vi "LSMcontroller_v66_improvedwfhandling.vi"() -> ()   [LabVIEW 2015] (continued)
                  frame #4 {
                    n2587 = call "tempconfigAO_seal.vi"("command"="get") -> ("Temp Config out"=w5912:T25)  [unwired: 1 in]
                    n2588 = Unbundle By Name(w5912) -> ("AO"=w5911:refnum<k21>[], "E_AO"=w5910:errorcluster[])
                    n2589 = call "tempconfigAI_seal.vi"("command"="get") -> ("Temp Config out"=w5899:T26)  [unwired: 1 in]
                    n2590 = call "configuration.vi"("command"="get") -> ("config out"=w5893:T11)  [unwired: 2 in, 1 out]
                    n2591 = Unbundle By Name(w5899) -> ("AI"=w5900:refnum<k21>, "E_AI"=w5901:errorcluster)
                    n2592 = Unbundle By Name(w5893) -> ("Device 1 sampleclock out"=w5890:tag, "Device 1 Starttrigger out"=w5889:tag)
                    n2593 = for {
                      tunnel: w5911 -> [w5916] mode=indexing
                      tunnel: w5910 -> [w5915] mode=indexing
                      tunnel: [w5914] -> w5906 mode=indexing
                      n2594 = call <vilib>:"DAQmx Stop Task.vi"("task/channels in"=w5916, "error in"=w5915) -> ("task out"=w5917:refnum<k21>, "error out"=w5918:errorcluster)  [unwired: 12 in]
                      n2595 = call <vilib>:"DAQmx Clear Task.vi"("task in"=w5917, "error in"=w5918) -> ("error out"=w5914:errorcluster)  [unwired: 13 in]
                    }
                    n2596 = call <vilib>:"DAQmx Stop Task.vi"("task/channels in"=w5900, "error in"=w5901) -> ("task out"=w5897:refnum<k21>, "error out"=w5896:errorcluster)  [unwired: 12 in]
                    n2597 = call <vilib>:"DAQmx Disconnect Terminals.vi"("source terminal"=tag "/Dev1/ai/SampleClock", "destination terminal"=w5890) -> ("error out"=w5887:errorcluster)  [unwired: 13 in]
                    n2598 = call <vilib>:"DAQmx Clear Task.vi"("task in"=w5897, "error in"=w5896) -> ("error out"=w5895:errorcluster)  [unwired: 13 in]
                    n2599 = call "tempconfigAO_seal.vi"("command"="get") -> ("Temp Config out"=w5907:T25)  [unwired: 1 in]
                    n2600 = Bundle By Name(cluster=w5907, "E_AO"=w5906) -> (w5905:T25)
                    n2601 = call "tempconfigAI_seal.vi"("command"="get") -> ("Temp Config out"=w5903:T26)  [unwired: 1 in]
                    n2602 = Bundle By Name(cluster=w5903, "E_AI"=w5895) -> (w5894:T26)
                    n2603 = call "tempconfigAO_seal.vi"("Temp Config in"=w5905, "command"="set") -> ()  [unwired: 1 out]
                    n2604 = call "tempconfigAI_seal.vi"("Temp Config in"=w5894, "command"="set") -> ()  [unwired: 1 out]
                    n2605 = call <vilib>:"DAQmx Disconnect Terminals.vi"("source terminal"=tag "/Dev1/ai/StartTrigger", "destination terminal"=w5889, "error in"=w5887) -> ()  [unwired: 12 in, 1 out]
                  }
                  frame #5 {
                    n2606 = call "zeropatch.vi"() -> ()  [unwired: 12 in]
                  }
                  frame #6 {
                    w5922 = T21 4 items=["no dialog", "OK message", "continue or stop message", "OK message + warnings", "continue/stop + warnings"] ("type of dialog (OK msg:1)")
                    n2607 = call "displayerrors.vi"() -> ("error IO"=w5921:errorcluster)
                    n2608 = call <vilib>:"Simple Error Handler.vi"("type of dialog (OK msg:1)"=w5922, "error in (no error)"=w5921) -> ("error out"=w5920:errorcluster)  [unwired: 3 in, 4 out]
                    n2609 = call <vilib>:"Clear Errors.vi"("error in (no error)"=w5920) -> ("error out"=w5919:errorcluster)  [unwired: 5 in, 1 out]
                    n2610 = call "seterrors.vi"("error IO"=w5919) -> ()
                  }
                }
              }
            }
          }
          event "readpatch": Value Change {
            n2611 = event-data() -> ()  [unwired: 1 in, 6 out]
            n2612 = local read "readpatch"() -> (w5923:bool)
            n2613 = case shown="True" w5923 {
              frame False {
              }
              frame True {
                n2614 = stacked-sequence {
                  seq-local: [w5924 _ _ _ _ _] -> [_ w5957 _ w6009 _ _]
                  frame #0 {
                    n2615 = stacked-sequence {
                      tunnel: [_ w5936 _] -> w5924
                      frame #0 {
                        n2616 = call "2pparameters.vi"("command"="get") -> ("params out"=w5929:T10)  [unwired: 1 in]
                        n2617 = Unbundle By Name(w5929) -> ("autoshutter"=w5930:bool)
                        n2618 = local read "OCchecked?"() -> (w5927:bool)
                        n2619 = call "sealtestwfparams.vi"("command"="set") -> ()  [unwired: 6 in, 1 out]
                        n2620 = case shown="False" w5927 {
                          frame False {
                            n2621 = One Button Dialog(message="Is the OC gain correct?", button name ("OK")="ok") -> (true=w5931:bool)
                            n2622 = local write "OCchecked?"(w5931) -> ()
                          }
                          frame True {
                          }
                        }
                        n2623 = case shown="True" w5930 {
                          frame False {
                          }
                          frame True {
                            n2624 = call "shuttercontrol.vi"("command"="close") -> ()  [unwired: 1 in, 1 out]
                          }
                        }
                        n2625 = call "allAI-temp.vi"("command"=enum16{"get", "set", "clear", "append"}."clear") -> ()  [unwired: 3 in, 2 out]
                      }
                      frame #1 {
                        n2626 = call "sealtestwfparams.vi"("command"="get") -> ("Params out"=w5942:T22)  [unwired: 6 in]
                        n2627 = Unbundle By Name(w5942) -> ("AO parameters"=w5940:T23)
                        n2628 = Index Array(array=w5940, index=1) -> (element=w5939:T24)
                        n2629 = call "generateRampedSquareWave_fromAOparameters.vi"("AO params"=w5939) -> ("Waveform"=w5935:waveform(dbl), "wflength"=w5936:i32)
                        n2630 = Build Array(w5935) -> (w5938:waveform(dbl)[])
                        n2631 = call "waveformssealtestbuffer.vi"("AO wf in"=w5938, "command"="set") -> ()  [unwired: 1 out]
                      }
                      frame #2 {
                        n2632 = local read "Vholding (mV)"() -> (w5945:sgl)
                        n2633 = local read "Current Clamp"() -> (w5951:bool)
                        n2634 = local read "Voltage Clamp"() -> (w5950:bool)
                        n2635 = local read "OCgain"() -> (w5946:sgl)
                        n2636 = local read "CC_ICgain"() -> (w5949:dbl)
                        n2637 = local read "holdon"() -> (w5944:bool)
                        n2638 = call "patchparameters.vi"("command"="get") -> ("Params out"=w5953:T13)  [unwired: 1 in]
                        n2639 = Bundle By Name(cluster=w5953, "VC"=w5950, "CC"=w5951, "CC_icg (pA/mv)"=w5949, "VC_icg (mV/mV)"=10.0, "OCG (mV/pA)"=w5946, "OVG (mV/mV)"=0.1, "Vhold (mV)"=w5945, "holdon"=w5944) -> (w5952:T13)
                        n2640 = call "patchparameters.vi"("Params in"=w5952, "command"="set") -> ()  [unwired: 1 out]
                      }
                    }
                  }
                  frame #1 {
                    w5956 = 2
                    n2641 = call "patchparameters.vi"("command"="get") -> ("Params out"=w5964:T13)  [unwired: 1 in]
                    n2642 = Unbundle By Name(w5964) -> ("holdon"=w5963:bool, "Vhold (mV)"=w5962:sgl, "CC_icg (pA/mv)"=w5970:sgl, "CC"=w5968:bool, "VC_icg (mV/mV)"=w5969:sgl)
                    n2643 = Select(t=w5970, s=w5968, f=w5969) -> (s? t:f=w5971:sgl)
                    n2644 = To Single Precision Float(number=0.001 ("y")) -> (single precision float=w5972:sgl)
                    n2645 = Compound Arithmetic op=MULTIPLY(w5962, w5971, w5972) -> (w5966:sgl)
                    n2646 = case shown="False" w5963 {
                      tunnel: w5966 -> [_ w5984]
                      tunnel: [0.0 w5984] -> w5959
                      frame False {
                      }
                      frame True {
                      }
                    }
                    n2647 = Greater Than 0?(x=w5956) -> (x > 0?=w5958:bool)
                    n2648 = case shown="True" w5958 {
                      tunnel: w5957 -> [_ w5973]
                      tunnel: w5956 -> [_ w5976]
                      frame False {
                      }
                      frame True {
                        n2649 = Initialize Array(sgl 0.0 ("element"), w5976, w5973) -> (w5974:sgl[][])
                        n2650 = call "allAI-temp.vi"("array in"=w5974, "command"=enum16{"get", "set", "clear", "append"}."set") -> ()  [unwired: 2 in, 2 out]
                      }
                    }
                    n2651 = flat-sequence {
                      tunnel: w5957 -> [w5980]
                      tunnel: w5957 -> [w5979]
                      tunnel: [w5979] -> w5961
                      tunnel: [w5978] -> w5960
                      tunnel: w5959 -> [w5978]
                      tunnel: w5961 -> [w5982]
                      tunnel: w5960 -> [w5981]
                      frame #0 {
                        n2652 = call "prepAI_sealtest.vi"("samples per channel"=w5980) -> ()  [unwired: 2 in]
                      }
                      frame #1 {
                        n2653 = call "prepAO_sealtest.vi"("Vhold"=w5981, "samples per channel"=w5982) -> ()  [unwired: 1 in]
                      }
                    }
                  }
                  frame #2 {
                    n2654 = stacked-sequence {
                      frame #0 {
                        n2655 = call "tempconfigAO.vi"("command"="get") -> ("Temp Config out"=w5988:T25)  [unwired: 1 in]
                        n2656 = Unbundle By Name(w5988) -> ("AO"=w5989:refnum<k21>[], "E_AO"=w5990:errorcluster[])
                        n2657 = for {
                          tunnel: w5989 -> [w5998] mode=indexing
                          tunnel: w5990 -> [w5997] mode=indexing
                          tunnel: [w5996] -> w5992 mode=indexing
                          tunnel: [w5995] -> w5993 mode=indexing
                          n2658 = call <vilib>:"DAQmx Start Task.vi"("task/channels in"=w5998, "error in"=w5997) -> ("task out"=w5996:refnum<k21>, "error out"=w5995:errorcluster)  [unwired: 12 in]
                        }
                        n2659 = call "tempconfigAO.vi"("command"="get") -> ("Temp Config out"=w5991:T25)  [unwired: 1 in]
                        n2660 = Bundle By Name(cluster=w5991, "AO"=w5992, "E_AO"=w5993) -> (w5994:T25)
                        n2661 = call "tempconfigAO.vi"("Temp Config in"=w5994, "command"="set") -> ()  [unwired: 1 out]
                      }
                      frame #1 {
                        n2662 = call "tempconfigAI.vi"("command"="get") -> ("Temp Config out"=w6000:T26)  [unwired: 1 in]
                        n2663 = Unbundle By Name(w6000) -> ("AI"=w6005:refnum<k21>, "E_AI"=w6006:errorcluster)
                        n2664 = call <vilib>:"DAQmx Start Task.vi"("task/channels in"=w6005, "error in"=w6006) -> ("task out"=w6007:refnum<k21>, "error out"=w6008:errorcluster)  [unwired: 12 in]
                        n2665 = call "tempconfigAI.vi"("command"="get") -> ("Temp Config out"=w6002:T26)  [unwired: 1 in]
                        n2666 = Bundle By Name(cluster=w6002, "AI"=w6007, "E_AI"=w6008) -> (w6004:T26)
                        n2667 = call "tempconfigAI.vi"("Temp Config in"=w6004, "command"="set") -> ()  [unwired: 1 out]
                      }
                    }
                  }
                  frame #3 {
                    n2668 = while {
                      tunnel: w6009 -> [w6010]
                      stop <- w6011 stop-if-true
                      n2669 = local read "readpatch"() -> (w6014:bool)
                      n2670 = Not(x=w6014) -> (.not. x?=w6013:bool)
                      n2671 = case shown="True" w6013 {
                        tunnel: w6010 -> [w6015 _]
                        frame False {
                          n2672 = stacked-sequence {
                            seq-local: [w6016 _ _ _ _ _] -> [_ w6025 _ w6048 w6095 w6114]
                            tunnel: w6015 -> [_ _ w6033 _ w6094 _]
                            frame #0 {
                              n2673 = call "patchparameters.vi"("command"="get") -> ("Params out"=w6023:T13)  [unwired: 1 in]
                              n2674 = local read "Vholding (mV)"() -> (w6020:sgl)
                              n2675 = Unbundle By Name(w6023) -> ("Vhold (mV)"=w6019:sgl, "holdon"=w6022:bool)
                              n2676 = local read "holdon"() -> (w6021:bool)
                              n2677 = Not Equal?(x=w6020, y=w6019) -> (x != y?=w6018:bool)
                              n2678 = Not Equal?(x=w6022, y=w6021) -> (x != y?=w6017:bool)
                              n2679 = Or(x=w6018, y=w6017) -> (x .or. y?=w6016:bool)
                            }
                            frame #1 {
                              n2680 = case shown="False" w6025 {
                                frame False {
                                }
                                frame True {
                                n2681 = local read "Vholding (mV)"() -> (w6028:sgl)
                                n2682 = local read "holdon"() -> (w6026:bool)
                                n2683 = call "patchparameters.vi"("command"="get") -> ("Params out"=w6029:T13)  [unwired: 1 in]
                                n2684 = Bundle By Name(cluster=w6029, "Vhold (mV)"=w6028, "holdon"=w6026) -> (w6027:T13)
                                n2685 = call "patchparameters.vi"("Params in"=w6027, "command"="set") -> ()  [unwired: 1 out]
                                }
                              }
                            }
                            frame #2 {
                              n2686 = call "tempconfigAI.vi"("command"="get") -> ("Temp Config out"=w6043:T26)  [unwired: 1 in]
                              n2687 = Unbundle By Name(w6043) -> ("AI"=w6042:refnum<k21>, "E_AI"=w6041:errorcluster)
                              n2688 = call-poly <vilib>:"DAQmx Read.vi"("task/channels in"=w6042, "number of samples per channel"=w6033, "timeout"=10.0, "error in"=w6041) -> ("task out"=w6037:refnum<k21>, "data"=w6034:i16[][], "error out"=w6046:errorcluster)  [unwired: 9 in]
                              n2689 = call "tempconfigAI.vi"("command"="get") -> ("Temp Config out"=w6038:T26)  [unwired: 1 in]
                              n2690 = Bundle By Name(cluster=w6038, "AI"=w6037, "E_AI"=w6046) -> (w6045:T26)
                              n2691 = To Single Precision Float(number=w6034) -> (single precision float=w6036:sgl[][])
                              n2692 = call "tempconfigAI.vi"("Temp Config in"=w6045, "command"="set") -> ()  [unwired: 1 out]
                              n2693 = call "allAI-temp.vi"("array in"=w6036, "command"=enum16{"get", "set", "clear", "append"}."set") -> ()  [unwired: 2 in, 2 out]
                            }
                            frame #3 {
                              n2694 = case shown="True" w6048 {
                                frame False {
                                }
                                frame True {
                                n2695 = call "tempconfigAO.vi"("command"="get") -> ("Temp Config out"=w6087:T25)  [unwired: 1 in]
                                n2696 = Unbundle By Name(w6087) -> ("AO"=w6086:refnum<k21>[], "E_AO"=w6085:errorcluster[])
                                n2697 = call "tempconfigAI.vi"("command"="get") -> ("Temp Config out"=w6074:T26)  [unwired: 1 in]
                                n2698 = Unbundle By Name(w6074) -> ("AI"=w6075:refnum<k21>, "E_AI"=w6076:errorcluster)
                                n2699 = for {
                                tunnel: w6086 -> [w6091] mode=indexing
                                tunnel: w6085 -> [w6090] mode=indexing
                                tunnel: [w6089] -> w6081 mode=indexing
                                n2700 = call <vilib>:"DAQmx Stop Task.vi"("task/channels in"=w6091, "error in"=w6090) -> ("task out"=w6092:refnum<k21>, "error out"=w6093:errorcluster)  [unwired: 12 in]
                                n2701 = call <vilib>:"DAQmx Clear Task.vi"("task in"=w6092, "error in"=w6093) -> ("error out"=w6089:errorcluster)  [unwired: 13 in]
                                }
                                n2702 = call <vilib>:"DAQmx Stop Task.vi"("task/channels in"=w6075, "error in"=w6076) -> ("task out"=w6072:refnum<k21>, "error out"=w6071:errorcluster)  [unwired: 12 in]
                                n2703 = call <vilib>:"DAQmx Clear Task.vi"("task in"=w6072, "error in"=w6071) -> ("error out"=w6070:errorcluster)  [unwired: 13 in]
                                n2704 = call "tempconfigAO.vi"("command"="get") -> ("Temp Config out"=w6082:T25)  [unwired: 1 in]
                                n2705 = Bundle By Name(cluster=w6082, "E_AO"=w6081) -> (w6080:T25)
                                n2706 = call "tempconfigAI.vi"("command"="get") -> ("Temp Config out"=w6078:T26)  [unwired: 1 in]
                                n2707 = Bundle By Name(cluster=w6078, "E_AI"=w6070) -> (w6069:T26)
                                n2708 = call "tempconfigAO.vi"("Temp Config in"=w6080, "command"="set") -> ()  [unwired: 1 out]
                                n2709 = call "tempconfigAI.vi"("Temp Config in"=w6069, "command"="set") -> ()  [unwired: 1 out]
                                }
                              }
                              n2710 = call "allAI-temp.vi"("command"=enum16{"get", "set", "clear", "append"}."get") -> ("array out"=w6052:sgl[][])  [unwired: 3 in, 1 out]
                              n2711 = call "tempconfigAI.vi"("command"="get") -> ("Temp Config out"=w6064:T26)  [unwired: 1 in]
                              n2712 = call "tempconfigAI.vi"("command"="get") -> ("Temp Config out"=w6066:T26)  [unwired: 1 in]
                              n2713 = Unbundle By Name(w6064) -> ("header"=w6062:dbl[])
                              n2714 = Unbundle By Name(w6066) -> ("header"=w6068:dbl[])
                              n2715 = Index Array(array=w6052, index (row) #1=1 ("index (row)"), index (row) #2=0 ("index (row)")) -> (element #1=w6050:sgl[], element #2=w6049:sgl[])  [unwired: 2 in]
                              n2716 = local read "OCgain"() -> (w6056:sgl)
                              n2717 = call "Unscaledtoscaled.vi"("Unscaled Data"=w6050, "Header Information"=w6062) -> ("Array"=w6061:sgl[])  [unwired: 1 in]
                              n2718 = call "Unscaledtoscaled.vi"("Unscaled Data"=w6049, "Header Information"=w6068) -> ("Array"=w6065:sgl[])  [unwired: 1 in]
                              n2719 = Multiply(x=w6061, y=0.1) -> (x*y=w6058:dbl[])
                              n2720 = Divide(x=w6065, y=w6056) -> (x/y=w6057:sgl[])
                              n2721 = Build Array(w6058, w6057) -> (w6060:dbl[][])
                              n2722 = Multiply(x=w6060, y=1000.0) -> (x*y=w6047:dbl[][])
                              n2723 = local write "Patch readout"(w6047) -> ()
                            }
                            frame #4 {
                              n2724 = case shown="True" w6095 {
                                tunnel: w6094 -> [_ w6096]
                                frame False {
                                }
                                frame True {
                                n2725 = call "patchparameters.vi"("command"="get") -> ("Params out"=w6100:T13)  [unwired: 1 in]
                                n2726 = Unbundle By Name(w6100) -> ("holdon"=w6099:bool, "Vhold (mV)"=w6098:sgl, "CC_icg (pA/mv)"=w6106:sgl, "CC"=w6104:bool, "VC_icg (mV/mV)"=w6105:sgl)
                                n2727 = Select(t=w6106, s=w6104, f=w6105) -> (s? t:f=w6107:sgl)
                                n2728 = To Single Precision Float(number=0.001 ("y")) -> (single precision float=w6108:sgl)
                                n2729 = Compound Arithmetic op=MULTIPLY(w6098, w6107, w6108) -> (w6102:sgl)
                                n2730 = case shown="True" w6099 {
                                tunnel: w6102 -> [_ w6113]
                                tunnel: [0.0 w6113] -> w6097
                                frame False {
                                }
                                frame True {
                                }
                                }
                                n2731 = flat-sequence {
                                tunnel: w6096 -> [w6109]
                                tunnel: w6097 -> [w6111]
                                tunnel: w6096 -> [w6110]
                                frame #0 {
                                n2732 = call "prepAI_sealtest.vi"("samples per channel"=w6109) -> ()  [unwired: 2 in]
                                }
                                frame #1 {
                                n2733 = call "prepAO_sealtest.vi"("Vhold"=w6111, "samples per channel"=w6110) -> ()  [unwired: 1 in]
                                }
                                }
                                }
                              }
                            }
                            frame #5 {
                              n2734 = case shown="True" w6114 {
                                frame False {
                                }
                                frame True {
                                n2735 = stacked-sequence {
                                frame #0 {
                                n2736 = call "tempconfigAO.vi"("command"="get") -> ("Temp Config out"=w6121:T25)  [unwired: 1 in]
                                n2737 = Unbundle By Name(w6121) -> ("AO"=w6120:refnum<k21>[], "E_AO"=w6119:errorcluster[])
                                n2738 = for {
                                tunnel: w6120 -> [w6128] mode=indexing
                                tunnel: w6119 -> [w6127] mode=indexing
                                tunnel: [w6126] -> w6117 mode=indexing
                                tunnel: [w6125] -> w6116 mode=indexing
                                n2739 = call <vilib>:"DAQmx Start Task.vi"("task/channels in"=w6128, "error in"=w6127) -> ("task out"=w6126:refnum<k21>, "error out"=w6125:errorcluster)  [unwired: 12 in]
                                }
                                n2740 = call "tempconfigAO.vi"("command"="get") -> ("Temp Config out"=w6118:T25)  [unwired: 1 in]
                                n2741 = Bundle By Name(cluster=w6118, "AO"=w6117, "E_AO"=w6116) -> (w6115:T25)
                                n2742 = call "tempconfigAO.vi"("Temp Config in"=w6115, "command"="set") -> ()  [unwired: 1 out]
                                }
                                frame #1 {
                                n2743 = call "tempconfigAI.vi"("command"="get") -> ("Temp Config out"=w6130:T26)  [unwired: 1 in]
                                n2744 = Unbundle By Name(w6130) -> ("AI"=w6135:refnum<k21>, "E_AI"=w6136:errorcluster)
                                n2745 = call <vilib>:"DAQmx Start Task.vi"("task/channels in"=w6135, "error in"=w6136) -> ("task out"=w6137:refnum<k21>, "error out"=w6138:errorcluster)  [unwired: 12 in]
                                n2746 = call "tempconfigAI.vi"("command"="get") -> ("Temp Config out"=w6132:T26)  [unwired: 1 in]
                                n2747 = Bundle By Name(cluster=w6132, "AI"=w6137, "E_AI"=w6138) -> (w6134:T26)
                                n2748 = call "tempconfigAI.vi"("Temp Config in"=w6134, "command"="set") -> ()  [unwired: 1 out]
                                }
                                }
                                }
                              }
                            }
                          }
                        }
                        frame True {
                        }
                      }
                      n2749 = local read "readpatch"() -> (w6012:bool)
                      n2750 = Not(x=w6012) -> (.not. x?=w6011:bool)
                    }
                  }
                  frame #4 {
                    n2751 = call "tempconfigAO.vi"("command"="get") -> ("Temp Config out"=w6164:T25)  [unwired: 1 in]
                    n2752 = Unbundle By Name(w6164) -> ("AO"=w6163:refnum<k21>[], "E_AO"=w6162:errorcluster[])
                    n2753 = call "configuration.vi"("command"="get") -> ("config out"=w6145:T11)  [unwired: 2 in, 1 out]
                    n2754 = call "tempconfigAI.vi"("command"="get") -> ("Temp Config out"=w6151:T26)  [unwired: 1 in]
                    n2755 = Unbundle By Name(w6145) -> ("Device 1 sampleclock out"=w6142:tag, "Device 1 Starttrigger out"=w6141:tag)
                    n2756 = Unbundle By Name(w6151) -> ("AI"=w6152:refnum<k21>, "E_AI"=w6153:errorcluster)
                    n2757 = for {
                      tunnel: w6163 -> [w6168] mode=indexing
                      tunnel: w6162 -> [w6167] mode=indexing
                      tunnel: [w6166] -> w6158 mode=indexing
                      n2758 = call <vilib>:"DAQmx Stop Task.vi"("task/channels in"=w6168, "error in"=w6167) -> ("task out"=w6169:refnum<k21>, "error out"=w6170:errorcluster)  [unwired: 12 in]
                      n2759 = call <vilib>:"DAQmx Clear Task.vi"("task in"=w6169, "error in"=w6170) -> ("error out"=w6166:errorcluster)  [unwired: 13 in]
                    }
                    n2760 = call <vilib>:"DAQmx Stop Task.vi"("task/channels in"=w6152, "error in"=w6153) -> ("task out"=w6149:refnum<k21>, "error out"=w6148:errorcluster)  [unwired: 12 in]
                    n2761 = call <vilib>:"DAQmx Disconnect Terminals.vi"("source terminal"=tag "/Dev1/ai/SampleClock", "destination terminal"=w6142) -> ("error out"=w6139:errorcluster)  [unwired: 13 in]
                    n2762 = call <vilib>:"DAQmx Clear Task.vi"("task in"=w6149, "error in"=w6148) -> ("error out"=w6147:errorcluster)  [unwired: 13 in]
                    n2763 = call "tempconfigAO.vi"("command"="get") -> ("Temp Config out"=w6159:T25)  [unwired: 1 in]
                    n2764 = Bundle By Name(cluster=w6159, "E_AO"=w6158) -> (w6157:T25)
                    n2765 = call "tempconfigAI.vi"("command"="get") -> ("Temp Config out"=w6155:T26)  [unwired: 1 in]
                    n2766 = Bundle By Name(cluster=w6155, "E_AI"=w6147) -> (w6146:T26)
                    n2767 = call "tempconfigAO.vi"("Temp Config in"=w6157, "command"="set") -> ()  [unwired: 1 out]
                    n2768 = call <vilib>:"DAQmx Disconnect Terminals.vi"("source terminal"=tag "/Dev1/ai/StartTrigger", "destination terminal"=w6141, "error in"=w6139) -> ()  [unwired: 12 in, 1 out]
                    n2769 = call "tempconfigAI.vi"("Temp Config in"=w6146, "command"="set") -> ()  [unwired: 1 out]
                  }
                  frame #5 {
                    w6173 = T21 4 items=["no dialog", "OK message", "continue or stop message", "OK message + warnings", "continue/stop + warnings"] ("type of dialog (OK msg:1)")
                    n2770 = call "displayerrors.vi"() -> ("error IO"=w6172:errorcluster)
                    n2771 = call "zeropatch.vi"() -> ()  [unwired: 12 in]
                    n2772 = call <vilib>:"Simple Error Handler.vi"("type of dialog (OK msg:1)"=w6173, "error in (no error)"=w6172) -> ("error out"=w6171:errorcluster)  [unwired: 3 in, 4 out]
                    n2773 = call <vilib>:"Clear Errors.vi"("error in (no error)"=w6171) -> ()  [unwired: 5 in, 2 out]
                  }
                }
              }
            }
          }
          event "Current Clamp": Value Change {
            n2774 = event-data() -> ()  [unwired: 1 in, 6 out]
            n2775 = local read "Current Clamp"() -> (w6178:bool)
            n2776 = property on="Vholding (mV)" class="DigNum (strict)"("Caption.Text"="Ihold (pA)") -> ()  [unwired: 2 in, 2 out]
            n2777 = Not(x=w6178) -> (.not. x?=w6177:bool)
            n2778 = property on="Voltage Clamp" class="Bool (strict)"("Value"=w6177) -> ()  [unwired: 2 in, 2 out]
            n2779 = One Button Dialog(message="Have you switched the HEKA to CC and changed the external input cable?", button name ("OK")="Ok") -> ()  [unwired: 1 out]
          }
          event "Voltage Clamp": Value Change {
            n2780 = event-data() -> ()  [unwired: 1 in, 6 out]
            n2781 = local read "Voltage Clamp"() -> (w6183:bool)
            n2782 = Not(x=w6183) -> (.not. x?=w6182:bool)
            n2783 = property on="Current Clamp" class="Bool (strict)"("Value"=w6182) -> ()  [unwired: 2 in, 2 out]
            n2784 = One Button Dialog(message="Have you switched the HEKA to VC and changed the external input cable?", button name ("OK")="Ok") -> ()  [unwired: 1 out]
            n2785 = property on="Vholding (mV)" class="DigNum (strict)"("Caption.Text"="Vhold (mV)") -> ()  [unwired: 2 in, 2 out]
          }
          event "OCgain": Value Change {
            n2786 = event-data() -> ()  [unwired: 1 in, 6 out]
            n2787 = local read "OCgain"() -> (w6186:sgl)
            n2788 = Less?(x=w6186, y=0.3) -> (x < y?=w6184:bool)
            n2789 = case shown="True" w6184 {
              frame False {
                w6187 = 10.0 items=["0.1"=10.0, "10"=0.1] ("CC_ICgain")
                n2790 = local write "CC_ICgain"(w6187) -> ()
              }
              frame True {
                w6188 = 0.1 items=["0.1"=10.0, "10"=0.1] ("CC_ICgain")
                n2791 = local write "CC_ICgain"(w6188) -> ()
              }
            }
          }
          event "holdon": Value Change {
            n2792 = event-data() -> ()  [unwired: 1 in, 6 out]
            n2793 = stacked-sequence {
              frame #0 {
                n2794 = local read "Vholding (mV)"() -> (w6192:sgl)
                n2795 = local read "holdon"() -> (w6189:bool)
                n2796 = call "patchparameters.vi"("command"="get") -> ("Params out"=w6193:T13)  [unwired: 1 in]
                n2797 = Bundle By Name(cluster=w6193, "Vhold (mV)"=w6192, "holdon"=w6189) -> (w6190:T13)
                n2798 = call "patchparameters.vi"("Params in"=w6190, "command"="set") -> ()  [unwired: 1 out]
              }
              frame #1 {
                n2799 = call "zeropatch.vi"() -> ()  [unwired: 12 in]
              }
            }
          }
          event "Vholding (mV)": Value Change {
            n2800 = event-data() -> ()  [unwired: 1 in, 6 out]
            n2801 = local read "holdon"() -> (w6195:bool)
            n2802 = case shown="True" w6195 {
              frame False {
              }
              frame True {
                n2803 = stacked-sequence {
                  frame #0 {
                    n2804 = local read "Vholding (mV)"() -> (w6198:sgl)
                    n2805 = local read "holdon"() -> (w6199:bool)
                    n2806 = call "patchparameters.vi"("command"="get") -> ("Params out"=w6200:T13)  [unwired: 1 in]
                    n2807 = Bundle By Name(cluster=w6200, "Vhold (mV)"=w6198, "holdon"=w6199) -> (w6196:T13)
                    n2808 = call "patchparameters.vi"("Params in"=w6196, "command"="set") -> ()  [unwired: 1 out]
                  }
                  frame #1 {
                    n2809 = call "zeropatch.vi"() -> ()  [unwired: 12 in]
                  }
                }
              }
            }
          }
          event "AI channels": Value Change {
            n2810 = event-data() -> ()  [unwired: 1 in, 6 out]
            n2811 = local read "CI channels"() -> (w6209:i32[])
            n2812 = local read "AI channels"() -> (w6210:i32[])
            n2813 = call "configuration.vi"("command"="get") -> ("config out"=w6203:T11)  [unwired: 2 in, 1 out]
            n2814 = Unbundle By Name(w6203) -> ("CI names"=w6204:string[], "AI names"=w6205:string[])
            n2815 = for {
              tunnel: w6209 -> [w6215] mode=indexing
              tunnel: w6204 -> [w6216]
              tunnel: [w6214] -> w6206 mode=indexing
              n2816 = Index Array(array=w6216, index=w6215) -> (element=w6214:string)
            }
            n2817 = for {
              tunnel: w6210 -> [w6212] mode=indexing
              tunnel: w6205 -> [w6213]
              tunnel: [w6211] -> w6207 mode=indexing
              n2818 = Index Array(array=w6213, index=w6212) -> (element=w6211:string)
            }
            n2819 = Build Array (concatenate)(w6206, w6207) -> (w6208:string[])
            n2820 = property on="image1list" class="Ring (strict)"("Strings []"=w6208) -> ()  [unwired: 2 in, 2 out]
            n2821 = property on="image2list" class="Ring (strict)"("Strings []"=w6208) -> ()  [unwired: 2 in, 2 out]
          }
          event "CI channels": Value Change {
            n2822 = event-data() -> ()  [unwired: 1 in, 6 out]
            n2823 = local read "CI channels"() -> (w6224:i32[])
            n2824 = local read "AI channels"() -> (w6225:i32[])
            n2825 = call "configuration.vi"("command"="get") -> ("config out"=w6218:T11)  [unwired: 2 in, 1 out]
            n2826 = Unbundle By Name(w6218) -> ("CI names"=w6219:string[], "AI names"=w6220:string[])
            n2827 = for {
              tunnel: w6224 -> [w6230] mode=indexing
              tunnel: w6219 -> [w6231]
              tunnel: [w6229] -> w6221 mode=indexing
              n2828 = Index Array(array=w6231, index=w6230) -> (element=w6229:string)
            }
            n2829 = for {
              tunnel: w6225 -> [w6227] mode=indexing
              tunnel: w6220 -> [w6228]
              tunnel: [w6226] -> w6222 mode=indexing
              n2830 = Index Array(array=w6228, index=w6227) -> (element=w6226:string)
            }
            n2831 = Build Array (concatenate)(w6221, w6222) -> (w6223:string[])
            n2832 = property on="image1list" class="Ring (strict)"("Strings []"=w6223) -> ()  [unwired: 2 in, 2 out]
            n2833 = property on="image2list" class="Ring (strict)"("Strings []"=w6223) -> ()  [unwired: 2 in, 2 out]
          }
          event "setdatdir": Value Change {
            n2834 = event-data() -> ()  [unwired: 1 in, 5 out]
            n2835 = case shown="True" "setdatdir" {
              frame False {
              }
              frame True {
                n2836 = stacked-sequence {
                  frame #0 {
                    n2837 = local read "data dir"() -> (w6233:path)
                    n2838 = call "File Dialog"("start path"=w6233, "prompt"="Please select data directory...") -> ("selected path"=w6235:path, "cancelled"=w6234:bool, "error out"=w6236:errorcluster)  [unwired: 10 in, 1 out]
                    n2839 = case shown="False" w6234 {
                      tunnel: w6235 -> [w6244 _]
                      tunnel: w6236 -> [w6241 w6247]
                      tunnel: [w6239 w6247] -> w6238
                      frame False {
                        n2840 = local write "data dir"(w6244) -> ()
                        n2841 = call "configuration.vi"("error in"=w6241, "command"="get") -> ("Error out"=w6240:errorcluster, "config out"=w6246:T11)  [unwired: 1 in]
                        n2842 = Bundle By Name(cluster=w6246, "master data dir"=w6244) -> (w6245:T11)
                        n2843 = call "configuration.vi"("error in"=w6240, "config in"=w6245, "command"="set") -> ("Error out"=w6239:errorcluster)  [unwired: 1 out]
                      }
                      frame True {
                      }
                    }
                    n2844 = local write "status"(w6238) -> ()
                  }
                  frame #1 {
                    n2845 = property on="setdatdir" class="Bool (strict)"("Value"=FALSE ("setdatdir")) -> ()  [unwired: 2 in, 2 out]
                  }
                }
              }
            }
          }
          event "Shutter": Value Change {
            n2846 = event-data() -> ()  [unwired: 1 in, 5 out]
            n2847 = case shown="False" "Shutter" {
              frame False {
                n2848 = call "shuttercontrol.vi"("command"="close") -> ()  [unwired: 1 in, 1 out]
              }
              frame True {
                n2849 = call "shuttercontrol.vi"("command"="open") -> ()  [unwired: 1 in, 1 out]
              }
            }
          }
          event "ROI": Value Change {
            n2850 = event-data() -> ()  [unwired: 1 in, 5 out]
            n2851 = local read "ROI"() -> (w6252:bool)
            n2852 = case shown="True" w6252 {
              frame False {
              }
              frame True {
                n2853 = stacked-sequence {
                  frame #0 {
                    n2854 = local read "Square pixels"() -> (w6269:bool)
                    n2855 = local read "square matrix"() -> (w6268:bool)
                    n2856 = local read "Vx-max ref"() -> (w6274:dbl)
                    n2857 = local read "Vx-min ref"() -> (w6273:dbl)
                    n2858 = local read "Vy-min ref"() -> (w6270:dbl)
                    n2859 = local read "ypixels ref"() -> (w6272:i32)
                    n2860 = local read "Vy-max ref"() -> (w6271:dbl)
                    n2861 = local read "xpixels ref"() -> (w6275:i32)
                    n2862 = local read "Angle ref"() -> (w6267:dbl)
                    n2863 = local read "Colormap"() -> (w6276:i32)
                    n2864 = call "2pparameters.vi"("command"="get") -> ("params out"=w6279:T10)  [unwired: 1 in]
                    n2865 = Bundle By Name(cluster=w6279, "Xpixels Img"=w6275, "Vx-min Img"=w6273, "VX-max Img"=w6274, "Ypixels Img"=w6272, "Vy-min Img"=w6270, "Vy-max Img"=w6271, "Colormap"=w6276, "square pixels"=w6269, "square matrix"=w6268, "Angle Img"=w6267) -> (w6278:T10)
                    n2866 = call "2pparameters.vi"("Params in"=w6278, "command"="set") -> ()  [unwired: 1 out]
                    n2867 = local read "Vx-max draw"() -> (w6259:dbl)
                    n2868 = local read "Angle drawing"() -> (w6266:dbl)
                    n2869 = local read "Vx-min draw"() -> (w6260:dbl)
                    n2870 = local read "Vy-min draw"() -> (w6263:dbl)
                    n2871 = local read "ypixels draw"() -> (w6261:dbl)
                    n2872 = local read "Vy-max draw"() -> (w6262:dbl)
                    n2873 = local read "Square pixels"() -> (w6264:bool)
                    n2874 = local read "square matrix"() -> (w6265:bool)
                    n2875 = local read "xpixels draw"() -> (w6258:dbl)
                    n2876 = local read "Colormap"() -> (w6257:i32)
                    n2877 = call "2pparameters.vi"("command"="get") -> ("params out"=w6254:T10)  [unwired: 1 in]
                    n2878 = Bundle By Name(cluster=w6254, "Xpixels"=w6258, "Vxminref"=w6260, "Vxmaxref"=w6259, "Ypixels"=w6261, "Vyminref"=w6263, "Vymaxref"=w6262, "Colormap"=w6257, "square pixels"=w6264, "square matrix"=w6265, "Angle draw"=w6266) -> (w6255:T10)
                    n2879 = call "2pparameters.vi"("Params in"=w6255, "command"="set") -> ()  [unwired: 1 out]
                  }
                  frame #1 {
                    n2880 = Current VI's Path() -> (path=w6290:path)
                    n2881 = Strip Path(path=w6290) -> (stripped path=w6291:path)  [unwired: 1 out]
                    n2882 = Build Path(base path=w6291, name or relative path="subVIs\\Image\\SetROI_v4.vi") -> (appended path=w6289:path)
                    n2883 = call <vilib>:"Set Busy.vi"() -> ("error out"=w6287:errorcluster)  [unwired: 10 in, 1 out]
                    n2884 = Open VI Reference(type specifier VI Refnum (for type only)=refnum<vi> refnum, vi path=w6289, error in (no error)=w6287) -> (vi reference=w6285:refnum<vi>, error out=w6283:errorcluster)  [unwired: 3 in]
                    n2885 = call-by-ref "?"(reference=w6285, error in=w6283) -> (reference out=w6284:refnum<vi>, error out=w6282:errorcluster)  [unwired: 1 in]
                    n2886 = Close Reference(reference=w6284, error in (no error)=w6282) -> (error out=w6286:errorcluster)
                    n2887 = call <vilib>:"Unset Busy.vi"("error in (no error)"=w6286) -> ()  [unwired: 10 in, 1 out]
                    n2888 = local write "status"(w6286) -> ()
                  }
                  frame #2 {
                    n2889 = call "2pparameters.vi"("command"="get") -> ("params out"=w6316:T10)  [unwired: 1 in]
                    n2890 = Unbundle By Name(w6316) -> ("Xpixels Img"=w6315:i32, "Vx-min Img"=w6314:dbl, "VX-max Img"=w6313:dbl, "Ypixels Img"=w6312:i32, "Vy-min Img"=w6311:dbl, "Vy-max Img"=w6310:dbl, "Colormap"=w6309:u16, "square pixels"=w6308:bool, "square matrix"=w6307:bool, "Angle Img"=w6306:dbl, "Drawing Mode"=w6305:u16)
                    n2891 = local write "xpixels ref"(w6315) -> ()
                    n2892 = local write "Vx-min ref"(w6314) -> ()
                    n2893 = local write "Vx-max ref"(w6313) -> ()
                    n2894 = local write "ypixels ref"(w6312) -> ()
                    n2895 = local write "Vy-min ref"(w6311) -> ()
                    n2896 = local write "Vy-max ref"(w6310) -> ()
                    n2897 = local write "Colormap"(w6309) -> ()
                    n2898 = local write "Square pixels"(w6308) -> ()
                    n2899 = local write "square matrix"(w6307) -> ()
                    n2900 = local write "Angle ref"(w6306) -> ()
                    n2901 = local write "ROI Type"(w6305) -> ()
                    n2902 = call "2pparameters.vi"("command"="get") -> ("params out"=w6299:T10)  [unwired: 1 in]
                    n2903 = Unbundle By Name(w6299) -> ("Xpixels"=w6293:i32, "Vxminref"=w6297:dbl, "Vxmaxref"=w6296:dbl, "Ypixels"=w6292:i32, "Vyminref"=w6295:dbl, "Vymaxref"=w6294:dbl, "Colormap"=w6300:u16, "square pixels"=w6301:bool, "square matrix"=w6302:bool, "Angle draw"=w6303:dbl, "Drawing Mode"=w6304:u16)
                    n2904 = local write "Vy-max draw"(w6294) -> ()
                    n2905 = local write "Angle drawing"(w6303) -> ()
                    n2906 = local write "Colormap"(w6300) -> ()
                    n2907 = local write "Square pixels"(w6301) -> ()
                    n2908 = local write "square matrix"(w6302) -> ()
                    n2909 = local write "ROI Type"(w6304) -> ()
                    n2910 = local write "xpixels draw"(w6293) -> ()
                    n2911 = local write "ypixels draw"(w6292) -> ()
                    n2912 = local write "Vx-min draw"(w6297) -> ()
                    n2913 = local write "Vx-max draw"(w6296) -> ()
                    n2914 = local write "Vy-min draw"(w6295) -> ()
                  }
                  frame #3 {
                    n2915 = property on="ROI" class="Bool (strict)"("Val(Sgnl)"=FALSE ("x/y scan")) -> ()  [unwired: 2 in, 2 out]
                  }
                }
              }
            }
          }
          event "Xdattype": Value Change {
            n2916 = event-data() -> ()  [unwired: 1 in, 1 out]
            n2917 = case shown="True" "Xdattype" {
              frame False {
              }
              frame True {
                n2918 = stacked-sequence {
                  frame #0 {
                    n2919 = Current VI's Path() -> (path=w6329:path)
                    n2920 = Strip Path(path=w6329) -> (stripped path=w6330:path)  [unwired: 1 out]
                    n2921 = Build Path(base path=w6330, name or relative path="subVIs\\Misc\\Changedataconfig.vi") -> (appended path=w6328:path)
                    n2922 = call <vilib>:"Set Busy.vi"() -> ("error out"=w6326:errorcluster)  [unwired: 10 in, 1 out]
                    n2923 = Open VI Reference(type specifier VI Refnum (for type only)=refnum<vi> refnum, vi path=w6328, error in (no error)=w6326) -> (vi reference=w6321:refnum<vi>, error out=w6323:errorcluster)  [unwired: 3 in]
                    n2924 = call-by-ref "?"(reference=w6321, error in=w6323) -> (reference out=w6325:refnum<vi>, error out=w6324:errorcluster)  [unwired: 12 in]
                    n2925 = Close Reference(reference=w6325, error in (no error)=w6324) -> (error out=w6320:errorcluster)
                    "status" <- w6320
                    n2926 = call <vilib>:"Unset Busy.vi"("error in (no error)"=w6320) -> ()  [unwired: 10 in, 1 out]
                  }
                  frame #1 {
                    n2927 = property on="Xdattype" class="Bool (strict)"("Val(Sgnl)"=FALSE ("x/y scan")) -> ()  [unwired: 2 in, 2 out]
                  }
                }
              }
            }
          }
          event "XautoOD": Value Change {
            n2928 = event-data() -> ()  [unwired: 1 in, 1 out]
            n2929 = case shown="True" "XautoOD" {
              frame False {
              }
              frame True {
                n2930 = stacked-sequence {
                  frame #0 {
                    n2931 = Current VI's Path() -> (path=w6342:path)
                    n2932 = Strip Path(path=w6342) -> (stripped path=w6343:path)  [unwired: 1 out]
                    n2933 = Build Path(base path=w6343, name or relative path="subVIs\\Misc\\ChangeautoODs.vi") -> (appended path=w6341:path)
                    n2934 = call <vilib>:"Set Busy.vi"() -> ("error out"=w6339:errorcluster)  [unwired: 10 in, 1 out]
                    n2935 = Open VI Reference(type specifier VI Refnum (for type only)=refnum<vi> refnum, vi path=w6341, error in (no error)=w6339) -> (vi reference=w6334:refnum<vi>, error out=w6336:errorcluster)  [unwired: 3 in]
                    n2936 = call-by-ref "?"(reference=w6334, error in=w6336) -> (reference out=w6338:refnum<vi>, error out=w6337:errorcluster)  [unwired: 12 in]
                    n2937 = Close Reference(reference=w6338, error in (no error)=w6337) -> (error out=w6333:errorcluster)
                    "status 2" <- w6333
                    n2938 = call <vilib>:"Unset Busy.vi"("error in (no error)"=w6333) -> ()  [unwired: 10 in, 1 out]
                  }
                  frame #1 {
                    n2939 = property on="XautoOD" class="Bool (strict)"("Val(Sgnl)"=FALSE ("x/y scan")) -> ()  [unwired: 2 in, 2 out]
                  }
                }
              }
            }
          }
          event "SetMan": Value Change {
            n2940 = event-data() -> ()  [unwired: 1 in, 1 out]
            n2941 = case shown="True" "SetMan" {
              frame False {
              }
              frame True {
                n2942 = stacked-sequence {
                  frame #0 {
                    w6346 = u16 0 items=["Rectangle", "Circle", "Freeform Boundary", "Freeform Interior"] ("ROI Type")
                    n2943 = local write "ROI Type"(w6346) -> ()
                    n2944 = local read "Square pixels"() -> (w6352:bool)
                    n2945 = case shown="True" w6352 {
                      frame False {
                        n2946 = local read "square matrix"() -> (w6353:bool)
                        n2947 = case shown="False" w6353 {
                          frame False {
                            "ypixels ref" <- "ypixels"
                            "xpixels ref" <- "xpixels"
                          }
                          frame True {
                            n2948 = local read "xpixels"() -> (w6358:i32)
                            n2949 = local read "ypixels"() -> (w6357:i32)
                            n2950 = Max & Min(x=w6358, y=w6357) -> (max(x,y)=w6356:i32)  [unwired: 1 out]
                            n2951 = local write "xpixels ref"(w6356) -> ()
                            n2952 = local write "ypixels ref"(w6356) -> ()
                          }
                        }
                      }
                      frame True {
                        n2953 = local read "square matrix"() -> (w6359:bool)
                        n2954 = case shown="False" w6359 {
                          frame False {
                            n2955 = local read "Vxmax"() -> (w6373:dbl)
                            n2956 = local read "Vx-min"() -> (w6372:dbl)
                            n2957 = local read "Vy-max"() -> (w6368:dbl)
                            n2958 = local read "Vy-min"() -> (w6369:dbl)
                            n2959 = Subtract(x=w6368, y=w6369) -> (x-y=w6370:dbl)
                            n2960 = Subtract(x=w6373, y=w6372) -> (x-y=w6371:dbl)
                            n2961 = Absolute Value(x=w6370) -> (abs(x)=w6361:dbl)
                            n2962 = Absolute Value(x=w6371) -> (abs(x)=w6362:dbl)
                            n2963 = Divide(x=w6362, y=w6361) -> (x/y=w6367:dbl)
                            n2964 = Greater Or Equal?(x=w6362, y=w6361) -> (x >= y?=w6360:bool)
                            n2965 = local read "xpixels"() -> (w6366:i32)
                            n2966 = local read "ypixels"() -> (w6363:i32)
                            n2967 = case shown="False" w6360 {
                              tunnel: w6367 -> [w6378 w6381]
                              tunnel: w6366 -> [w6375 _]
                              tunnel: [w6375 w6380] -> w6365
                              tunnel: [w6374 w6379] -> w6364
                              tunnel: w6363 -> [_ w6379]
                              frame False {
                                n2968 = To Double Precision Float(number=w6375) -> (double precision float=w6377:dbl)
                                n2969 = Divide(x=w6377, y=w6378) -> (x/y=w6376:dbl)
                                n2970 = To Long Integer(number=w6376) -> (32bit integer=w6374:i32)
                              }
                              frame True {
                                n2971 = To Double Precision Float(number=w6379) -> (double precision float=w6383:dbl)
                                n2972 = Multiply(x=w6383, y=w6381) -> (x*y=w6382:dbl)
                                n2973 = To Long Integer(number=w6382) -> (32bit integer=w6380:i32)
                              }
                            }
                            n2974 = local write "ypixels ref"(w6364) -> ()
                            n2975 = local write "xpixels ref"(w6365) -> ()
                          }
                          frame True {
                          }
                        }
                      }
                    }
                    "Vx-max ref" <- "Vxmax"
                    "Vx-min ref" <- "Vx-min"
                    "Vy-max ref" <- "Vy-max"
                    "Vy-min ref" <- "Vy-min"
                    "Angle ref" <- "Angle"
                  }
                  frame #1 {
                    n2976 = property on="SetMan" class="Bool (strict)"("Val(Sgnl)"=FALSE ("Value (Signaling)")) -> ()  [unwired: 2 in, 2 out]
                  }
                }
              }
            }
          }
          event "SetMan 2": Value Change {
            n2977 = event-data() -> ()  [unwired: 1 in, 1 out]
            n2978 = case shown="True" "SetMan 2" {
              frame False {
              }
              frame True {
                n2979 = stacked-sequence {
                  frame #0 {
                    n2980 = local write "Vx-ref"("Vx") -> ()
                    n2981 = local write "Vy-ref"("Vy") -> ()
                  }
                  frame #1 {
                    n2982 = property on="SetMan 2" class="Bool (strict)"("Val(Sgnl)"=FALSE ("Value (Signaling)")) -> ()  [unwired: 2 in, 2 out]
                  }
                }
              }
            }
          }
          event "Reset Coords": Value Change {
            n2983 = event-data() -> ("NewVal"=w6389:bool)  [unwired: 1 in, 5 out]
            n2984 = case shown="True" w6389 {
              frame False {
              }
              frame True {
                n2985 = stacked-sequence {
                  frame #0 {
                    n2986 = local write "xpixels"(256 ("xpixels")) -> ()
                    n2987 = local write "ypixels"(256 ("ypixels")) -> ()
                    n2988 = local write "Vxmax"(9.0 ("Vx-max")) -> ()
                    n2989 = local write "Vx-min"(-9.0 ("Vx-min")) -> ()
                    n2990 = local write "Vy-max"(9.0 ("Vy-max")) -> ()
                    n2991 = local write "Vy-min"(-9.0 ("Vy-min")) -> ()
                    n2992 = local write "Angle"(0.0 ("Angle")) -> ()
                  }
                  frame #1 {
                    n2993 = property on="Reset Coords" class="Bool (strict)"("Value"=FALSE ("TROI")) -> ()  [unwired: 2 in, 2 out]
                  }
                }
              }
            }
          }
          event "TROI": Value Change {
            n2994 = event-data() -> ()  [unwired: 1 in, 1 out]
            n2995 = case shown="True" "TROI" {
              frame False {
              }
              frame True {
                n2996 = stacked-sequence {
                  frame #0 {
                    n2997 = local read "Vy-min ref"() -> (w6403:dbl)
                    n2998 = local read "Vy-max ref"() -> (w6402:dbl)
                    n2999 = local read "Vx-max ref"() -> (w6400:dbl)
                    n3000 = local read "Vx-min ref"() -> (w6401:dbl)
                    n3001 = local read "ypixels ref"() -> (w6405:i32)
                    n3002 = local read "xpixels ref"() -> (w6404:i32)
                    n3003 = local read "Angle ref"() -> (w6399:dbl)
                    n3004 = local write "Angle"(w6399) -> ()
                    n3005 = local write "xpixels"(w6404) -> ()
                    n3006 = local write "Vy-min"(w6403) -> ()
                    n3007 = local write "Vy-max"(w6402) -> ()
                    n3008 = local write "Vx-min"(w6401) -> ()
                    n3009 = local write "ypixels"(w6405) -> ()
                    n3010 = local write "Vxmax"(w6400) -> ()
                  }
                  frame #1 {
                    n3011 = property on="TROI" class="Bool (strict)"("Value"=FALSE ("TROI")) -> ()  [unwired: 2 in, 2 out]
                  }
                }
              }
            }
          }
          event "TROI 2": Value Change {
            n3012 = event-data() -> ()  [unwired: 1 in, 1 out]
            n3013 = case shown="True" "TROI 2" {
              frame False {
              }
              frame True {
                n3014 = stacked-sequence {
                  frame #0 {
                    n3015 = local read "Vx-ref"() -> (w6408:dbl)
                    n3016 = local read "Vy-ref"() -> (w6409:dbl)
                    n3017 = local write "Vx"(w6408) -> ()
                    n3018 = local write "Vy"(w6409) -> ()
                  }
                  frame #1 {
                    n3019 = property on="TROI 2" class="Bool (strict)"("Value"=FALSE ("TROI")) -> ()  [unwired: 2 in, 2 out]
                  }
                }
              }
            }
          }
          event "Square pixels": Value Change {
            n3020 = event-data() -> ()  [unwired: 1 in, 1 out]
            n3021 = case shown="True" "Square pixels" {
              frame False {
              }
              frame True {
                n3022 = property on="square matrix" class="Bool (strict)"("Value"=FALSE ("square matrix")) -> ()  [unwired: 2 in, 2 out]
                n3023 = property on="Square pixels" class="Bool (strict)"("Value"=TRUE ("square matrix")) -> ()  [unwired: 2 in, 2 out]
              }
            }
          }
          event "square matrix": Value Change {
            n3024 = event-data() -> ()  [unwired: 1 in, 1 out]
            n3025 = case shown="True" "square matrix" {
              frame False {
              }
              frame True {
                n3026 = property on="square matrix" class="Bool (strict)"("Value"=TRUE ("square matrix")) -> ()  [unwired: 2 in, 2 out]
                n3027 = property on="Square pixels" class="Bool (strict)"("Value"=FALSE ("square matrix")) -> ()  [unwired: 2 in, 2 out]
              }
            }
          }
          event "up", "downright", "down", "downleft", "right", "left", "upright", "upleft": Value Change {
            n3028 = event-data() -> ()  [unwired: 1 in, 6 out]
            n3029 = local read "downright"() -> (w6422:bool)
            n3030 = local read "downleft"() -> (w6424:bool)
            n3031 = local read "upright"() -> (w6420:bool)
            n3032 = local read "upleft"() -> (w6418:bool)
            n3033 = local read "down"() -> (w6423:bool)
            n3034 = local read "right"() -> (w6421:bool)
            n3035 = local read "left"() -> (w6425:bool)
            n3036 = local read "up"() -> (w6419:bool)
            n3037 = Compound Arithmetic op=OR(w6418, w6419, w6420, w6421, w6422, w6423, w6424, w6425) -> (w6417:bool)
            n3038 = case shown="True" w6417 {
              frame False {
              }
              frame True {
                n3039 = stacked-sequence {
                  frame #0 {
                    n3040 = local read "downright"() -> (w6427:bool)
                    n3041 = local read "downleft"() -> (w6429:bool)
                    n3042 = local read "BigSmall"() -> (w6426:bool)
                    n3043 = local read "upright"() -> (w6431:bool)
                    n3044 = local read "upleft"() -> (w6434:bool)
                    n3045 = local read "down"() -> (w6430:bool)
                    n3046 = local read "right"() -> (w6432:bool)
                    n3047 = local read "left"() -> (w6428:bool)
                    n3048 = local read "up"() -> (w6433:bool)
                    n3049 = call "movestageparams.vi"("command"="get") -> ("Params out"=w6437:T20)  [unwired: 1 in]
                    n3050 = Bundle By Name(cluster=w6437, "upleft"=w6434, "up"=w6433, "upright"=w6431, "right"=w6432, "downright"=w6427, "down"=w6430, "downleft"=w6429, "left"=w6428, "Bigsmall"=w6426) -> (w6438:T20)
                    n3051 = call "movestageparams.vi"("Params in"=w6438, "command"="set") -> ()  [unwired: 1 out]
                  }
                  frame #1 {
                    n3052 = disable-structure shown="Disabled" {
                      frame Disabled {
                        n3053 = call "configuration.vi"("command"="get") -> ("config out"=w6441:T11)  [unwired: 2 in, 1 out]
                        n3054 = in-place {
                          n3055 = in-place-cluster #45(w6441) -> ()  [unwired: 2 out]
                          n3056 = in-place-cluster #45("StageL"="StageL", "StageS"="StageS") -> (w6439:T11)
                        }
                        n3057 = call "configuration.vi"("config in"=w6439, "command"="set") -> ()  [unwired: 1 in, 2 out]
                      }
                      frame Enabled {
                      }
                    }
                  }
                  frame #2 {
                    n3058 = call "movestage.vi"() -> ()  [unwired: 12 in]
                  }
                  frame #3 {
                    w6445 = FALSE ("OK Button")
                    w6446 = FALSE ("OK Button")
                    n3059 = property on="down" class="Bool (strict)"("Value"=w6446) -> ()  [unwired: 2 in, 2 out]
                    n3060 = property on="up" class="Bool (strict)"("Value"=w6446) -> ()  [unwired: 2 in, 2 out]
                    n3061 = property on="right" class="Bool (strict)"("Value"=w6446) -> ()  [unwired: 2 in, 2 out]
                    n3062 = property on="left" class="Bool (strict)"("Value"=w6446) -> ()  [unwired: 2 in, 2 out]
                    n3063 = property on="upright" class="Bool (strict)"("Value"=w6445) -> ()  [unwired: 2 in, 2 out]
                    n3064 = property on="downleft" class="Bool (strict)"("Value"=w6445) -> ()  [unwired: 2 in, 2 out]
                    n3065 = property on="downright" class="Bool (strict)"("Value"=w6445) -> ()  [unwired: 2 in, 2 out]
                    n3066 = property on="upleft" class="Bool (strict)"("Value"=w6445) -> ()  [unwired: 2 in, 2 out]
                  }
                }
              }
            }
          }
          event "finite samples": Value Change {
            n3067 = event-data() -> ("NewVal"=w6447:bool)  [unwired: 1 in]
            n3068 = flat-sequence {
              tunnel: w6447 -> [w6448]
              frame #0 {
                n3069 = case shown="True" w6448 {
                  frame False {
                    w6449 = FALSE ("wavdet")
                    n3070 = property on="continuous" class="Bool (strict)"("Value"=TRUE ("continuous for display")) -> ()  [unwired: 2 in, 2 out]
                    n3071 = property on="wavdet" class="Bool (strict)"("Value"=w6449) -> ()  [unwired: 2 in, 2 out]
                    n3072 = property on="save\ndata" class="Bool (strict)"("Value"=w6449) -> ()  [unwired: 2 in, 2 out]
                    n3073 = property on="# of frames" class="DigNum (strict)"("DisabledEnum"=T7."Disabled and Grayed Out" ("Disabled")) -> ()  [unwired: 2 in, 2 out]
                    n3074 = property on="save\ndata" class="Bool (strict)"("DisabledEnum"=T7."Disabled and Grayed Out" ("Disabled")) -> ()  [unwired: 2 in, 2 out]
                    "Save tab" <- enum32{"withsave", "withoutsave"}."withsave" ("Save tab")
                  }
                  frame True {
                    w6456 = FALSE ("continuous for display")
                    n3075 = property on="continuous" class="Bool (strict)"("Value"=w6456) -> ()  [unwired: 2 in, 2 out]
                    n3076 = property on="wavdet" class="Bool (strict)"("Value"=w6456) -> ()  [unwired: 2 in, 2 out]
                    n3077 = local write "Save tab"(enum32{"withsave", "withoutsave"}."withsave" ("Save tab")) -> ()
                    n3078 = property on="save\ndata" class="Bool (strict)"("DisabledEnum"=T7."Enabled" ("Disabled")) -> ()  [unwired: 2 in, 2 out]
                    n3079 = property on="save\ndata" class="Bool (strict)"("Value"=TRUE ("save\ndata")) -> ()  [unwired: 2 in, 2 out]
                    n3080 = property on="# of frames" class="DigNum (strict)"("DisabledEnum"=T7."Enabled" ("Disabled")) -> ()  [unwired: 2 in, 2 out]
                  }
                }
              }
              frame #1 {
                n3081 = local read "finite samples"() -> (w6465:bool)
                n3082 = local read "continuous"() -> (w6464:bool)
                n3083 = local read "wavdet"() -> (w6463:bool)
                n3084 = call "2pparameters.vi"("command"="get") -> ("params out"=w6459:T10)  [unwired: 1 in]
                n3085 = Bundle By Name(cluster=w6459, "finite"=w6465, "cont"=w6464, "wavdet"=w6463) -> (w6462:T10)
                n3086 = call "2pparameters.vi"("Params in"=w6462, "command"="set") -> ()  [unwired: 1 out]
              }
            }
          }
          event "continuous": Value Change {
            n3087 = event-data() -> ("NewVal"=w6466:bool)  [unwired: 1 in]
            n3088 = flat-sequence {
              tunnel: w6466 -> [w6467]
              frame #0 {
                n3089 = case shown="True" w6467 {
                  frame False {
                    n3090 = property on="finite samples" class="Bool (strict)"("Value"=TRUE ("finite samples for recording")) -> ()  [unwired: 2 in, 2 out]
                    n3091 = property on="save\ndata" class="Bool (strict)"("Value"=TRUE ("save\ndata")) -> ()  [unwired: 2 in, 2 out]
                    n3092 = property on="wavdet" class="Bool (strict)"("Value"=FALSE ("wavdet")) -> ()  [unwired: 2 in, 2 out]
                    n3093 = local write "Save tab"(enum32{"withsave", "withoutsave"}."withsave" ("Save tab")) -> ()
                    n3094 = property on="# of frames" class="DigNum (strict)"("DisabledEnum"=T7."Enabled" ("Disabled")) -> ()  [unwired: 2 in, 2 out]
                    n3095 = property on="save\ndata" class="Bool (strict)"("DisabledEnum"=T7."Enabled" ("Disabled")) -> ()  [unwired: 2 in, 2 out]
                  }
                  frame True {
                    w6474 = FALSE ("finite samples for recording")
